vi "SubGenerateListToOrder.vi"(8 "error in (no error)":errorcluster, 11 "SolutionBuilder in":refnum<class "SolutionBuilder.lvclass">) -> (0 "error out":errorcluster, 1 "Ordering map":T1, 3 "SolutionBuilder out":refnum<class "SolutionBuilder.lvclass">)   [LabVIEW 2020, in "SolutionBuilder.lvlib" / "SolutionBuilder.lvclass"]
uses:
  SolutionBuilder.lvclass
  OrderingMap.ctl
  ProjectItem/ProjectItem.lvclass
  SolutionBuilder.lvclass/SolutionBuilder.ctl
  <vilib>/Utility/miscctls.llb/LVMapReplaceAction.ctl
  be8949a1-daf6-466d-868e-55db06778a0f.vi
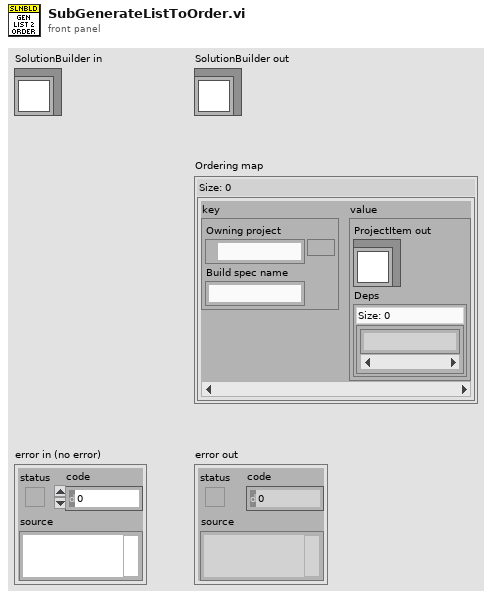
[diagram p1: front panel]
types:
  T1 = typedef "SolutionBuilder.lvlib/SolutionBuilder.lvclass/OrderingMap.ctl" = map{cluster{"Owning project":path, "Build spec name":string}, cluster{"ProjectItem out":refnum<class "ProjectItem.lvclass">, "Deps":set{string}}}
  T2 = typedef "SolutionBuilder.lvlib/SolutionBuilder.lvclass/ProjectItemMap.ctl" = map{path, refnum<class "ProjectItem.lvclass">[]}
  T3 = typedef "LVMapReplaceAction.ctl" = enum32{"Modify Entry only if found", "Add or Modify Entry", "Delete Entry"}
  T4 = cluster{"Owning project":path, "Build spec name":string}
  T5 = cluster{"ProjectItem out":refnum<class "ProjectItem.lvclass">, "Deps":set{string}}
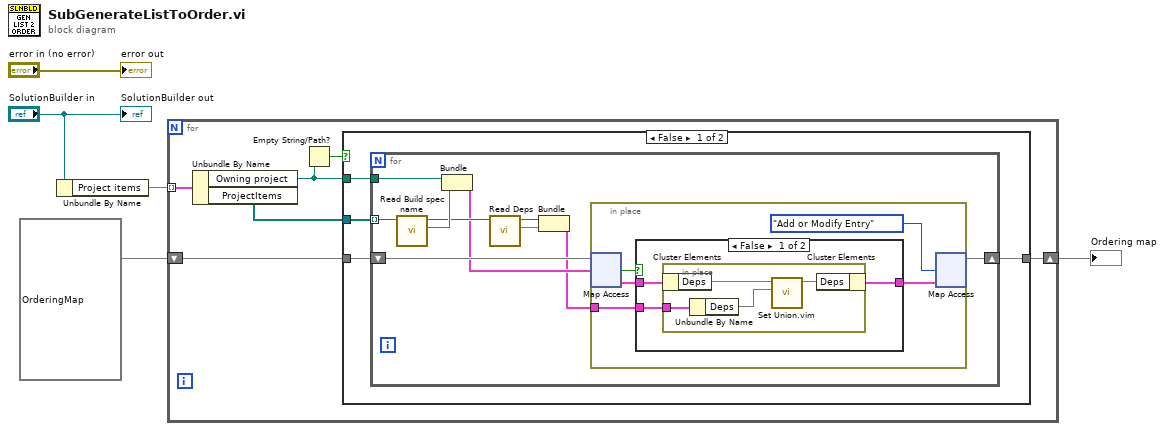
[diagram p0: block diagram]
diagram:
  n1 = Unbundle By Name("SolutionBuilder in") -> ("Project items"=w4:T2)
  n2 = for {
    tunnel: w4 -> [w11] mode=indexing
    shift-right: [w6] -> w2
    shift-left: T1 {} ("Ordering map") -> [w7]
    n3 = Unbundle By Name(w11) -> ("Owning project"=w10:path, "ProjectItems"=w8:refnum<class "ProjectItem.lvclass">[])
    n4 = Empty String/Path?(string/path=w10) -> (empty?=w9:bool)
    n5 = case shown="False" w9 {
      tunnel: w10 -> [w14 _]
      tunnel: w8 -> [w15 _]
      tunnel: w7 -> [w13 w39]
      tunnel: [w12 w39] -> w6
      frame False {
        n6 = for {
          tunnel: w15 -> [w25] mode=indexing
          tunnel: w14 -> [w20]
          shift-right: [w16] -> w12
          shift-left: w13 -> [w19]
          n7 = call-dynamic "Read Build spec name.vi"("ProjectItem in"=w25) -> ("Build spec name"=w24:string, "ProjectItem out"=w23:refnum<class "ProjectItem.lvclass">)  [unwired: 9 in]
          n8 = Bundle("Owning project"=w20, "Build spec name"=w24) -> (w18:T4)  [unwired: 1 in]
          n9 = call-dynamic "Read Deps.vi"("ProjectItem in"=w23) -> ("Deps"=w21:set{string}, "ProjectItem out"=w22:refnum<class "ProjectItem.lvclass">)  [unwired: 9 in]
          n10 = Bundle("ProjectItem out"=w22, "Deps"=w21) -> (w17:T5)  [unwired: 1 in]
          n11 = in-place {
            in-place-border: w17 -> [w29]
            n12 = in-place-map #1(w19, w18) -> (w26:T5, w30:bool)  [unwired: 1 in]
            n13 = case shown="False" w30 {
              tunnel: w29 -> [w32 w38]
              tunnel: [w31 w38] -> w28
              tunnel: w26 -> [w33 _]
              frame False {
                n14 = in-place {
                  in-place-border: w32 -> [w37]
                  n15 = in-place-cluster #2(w33) -> ("Deps"=w36:set{string})
                  n16 = Unbundle By Name(w37) -> ("Deps"=w35:set{string})
                  n17 = call "Set Union.vim"("set 2"=w35, "set 1"=w36) -> ("union"=w34:set{string})  [unwired: 9 in]
                  n18 = in-place-cluster #2("Deps"=w34) -> (w31:T5)
                }
              }
              frame True {
              }
            }
            n19 = in-place-map #1(w28, LVMapReplaceAction."Add or Modify Entry" ("action")) -> (w16:T1)  [unwired: 2 out]
          }
        }
      }
      frame True {
      }
    }
  }
  "Ordering map" <- w2
  "SolutionBuilder out" <- "SolutionBuilder in"
  "error out" <- "error in (no error)"
